vi "sccusess1.vi"() -> ()   [LabVIEW 2024]
panel:
  in  "stop":bool
  in  "count":i32
  out "counter":i32
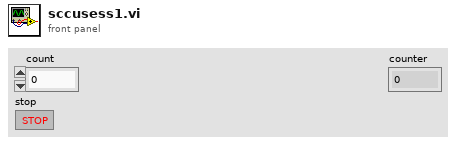
[diagram p1: front panel]
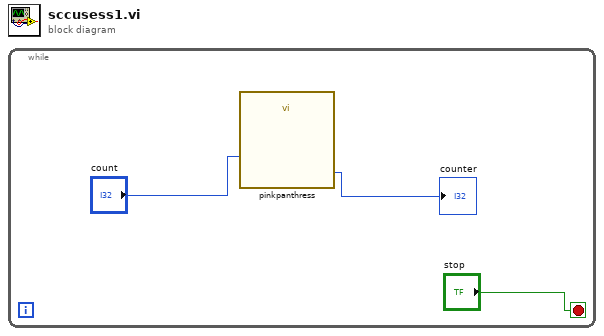
[diagram p0: block diagram]
diagram:
  n1 = while {
    stop <- "stop" stop-if-true
    n2 = call "pinkpanthress"("count"="count") -> ("counter"=→"counter":i32)  [unwired: 10 in]
  }
